vi "Edgertronic-:get_saved_settings copy.vi"(5 "Setup":T2={"URL"="130.64.16.195", "remote port"=80, "mode (standard)"=enum."Standard"}) -> (0 "error out":errorcluster, 1 "Saved Settings:":T1={"Connection Information:"="", "Requested Genlock "="20140911165611", "Min Frame Clocks "="20140911165611", "Is Seq Clk Freq "="20140911165611", "Pretrigger Frames "="20140911165611", "Duration "="20140911165611", "Overclock "="20140911165611", "Requested Horizontal "="20140911165611", "Frames "="20140911165611", "Requested Pretrigger "="20140911165611", "Words per Frame "="20140911165611", "Buffer End "="20140911165611", "Clocks per Frame  "="20140911165611", "Requested Duration "="20140911165611", "Pretrigger "="20140911165611", "Post-trigger Frames "="20140911165611", "Vertical "="20140911165611", "Requested Vertical "="20140911165611", "Reqested Frame Rate "="20140911165611", "Frame Rate "="20140911165611", "Horizontal "="20140911165611", "Clocks per Exposure "="20140911165611", "Digital Gain "="20140911165611", "Exposure "="20140911165611", "Genlock "="20140911165611", "Analog Gain "="20140911165611", "Subsample "="20140911165611", "Requested Exposure "="20140911165611", "Iso "="20140911165611", "Requested Overclock "="20140911165611", "Requested Subsample "="20140911165611", "Requested Iso"="20140911165611"}, 2 "data out":string="HTTP/1.0 200 OK\r\nContent-Type: text/html; charset=utf-8\r\nContent-Length: 313\r\nConnection: close\r\nDate: Tue, 16 Jun 2015 13:54:12 GMT\r\nServer: lighttpd/1.4.11 (edgertonic slow motion camera)\r\n\r\n{\"build_date\": \"20150112\", \"sw_build_date\": \"20140911165611\", \"fpga_initialized\": 1, \"hardware_revision\": 6, \"model_number\": 1, \"home_dir\": \"/home/root/ss-web\", \"ir_filter\": 1, \"mac_addr\": \"00:1B:C5:09:61:4D\", \"serial_console_enabled\": false, \"serial_number\": 333, \"fpga_version\": 70, \"hardware_configuration\": 1}")   [LabVIEW 2012]
doc: "This VI returns the values of the default settings."
panel:
  in  "GET Cmd":string="/get_saved_settings"
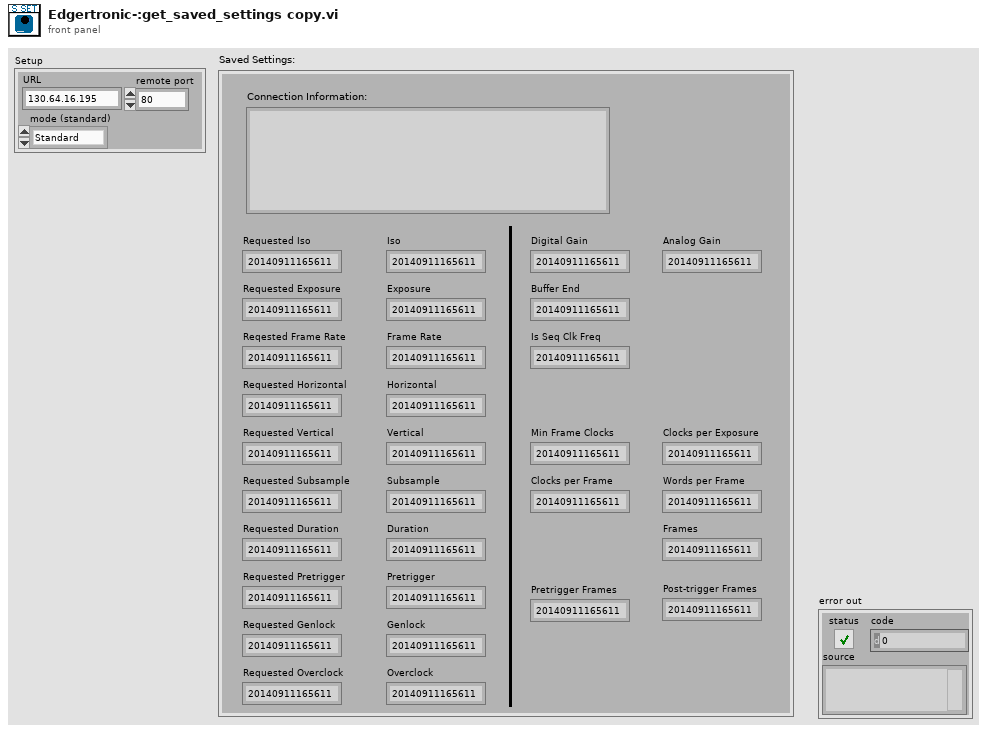
[diagram p1: front panel]
types:
  T1 = cluster{"Connection Information:":string, "Requested Genlock ":string, "Min Frame Clocks ":string, "Is Seq Clk Freq ":string, "Pretrigger Frames ":string, "Duration ":string, "Overclock ":string, "Requested Horizontal ":string, "Frames ":string, "Requested Pretrigger ":string, "Words per Frame ":string, "Buffer End ":string, "Clocks per Frame  ":string, "Requested Duration ":string, "Pretrigger ":string, "Post-trigger Frames ":string, "Vertical ":string, "Requested Vertical ":string, "Reqested Frame Rate ":string, "Frame Rate ":string, "Horizontal ":string, "Clocks per Exposure ":string, "Digital Gain ":string, "Exposure ":string, "Genlock ":string, "Analog Gain ":string, "Subsample ":string, "Requested Exposure ":string, "Iso ":string, "Requested Overclock ":string, "Requested Subsample ":string, "Requested Iso":string}
  T2 = cluster{"URL":string, "remote port":u16, "mode (standard)":enum16{"Standard", "Buffered", "CRLF", "Immediate"}}
  T3 = cluster{"Parameter":string, "Parameter 2":string, "Parameter 3":string, "Parameter 4":string, "Parameter 5":string, "Parameter 6":string, "Parameter 7":string, "Parameter 8":string, "Parameter 9":string, "Parameter 10":string, "Parameter 11":string, "Parameter 12":string, "Parameter 13":string, "Parameter 14":string, "Parameter 15":string, "Parameter 16":string, "Parameter 17":string, "Parameter 18":string, "Parameter 19":string, "Parameter 20":string, "Parameter 21":string, "Parameter 22":string, "Parameter 23":string, "Parameter 24":string, "Parameter 25":string, "Parameter 26":string, "Parameter 27":string, "Parameter 28":string, "Parameter 29":string, "Parameter 30":string, "Parameter 31":string, string, string, string, string, string}
  T4 = cluster{"[0]":string, "[1]":string, "[2]":string, "[3]":string, "[4]":string, "[5]":string, "[6]":string, "[7]":string, "[8]":string, "[9]":string, "[10]":string, "[11]":string, "[12]":string, "[13]":string, "[14]":string, "[15]":string, "[16]":string, "[17]":string, "[18]":string, "[19]":string, "[20]":string, "[21]":string, "[22]":string, "[23]":string, "[24]":string, "[25]":string, "[26]":string, "[27]":string, "[28]":string, "[29]":string, "[30]":string, "[31]":string, "[32]":string, "[33]":string, "[34]":string, "[35]":string}
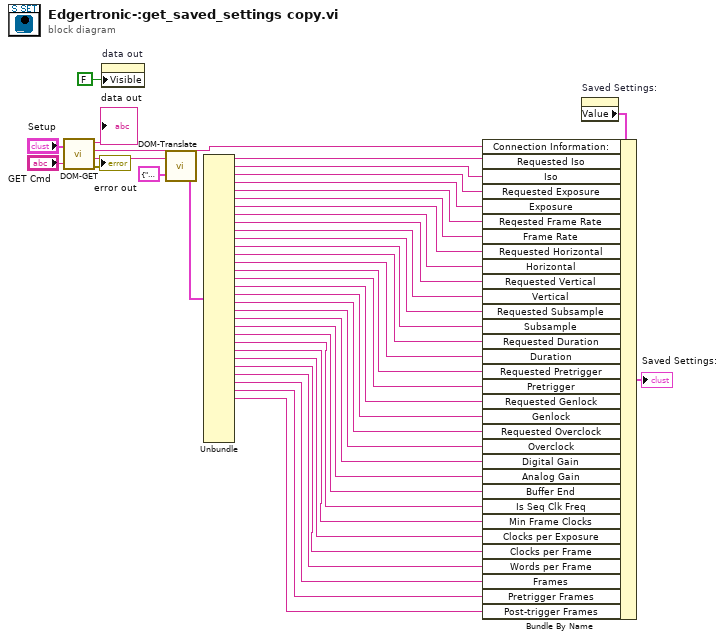
[diagram p0: block diagram]
diagram:
  n1 = call <userlib>:"DOM-GET.vi"("Setup"="Setup", "GET Command"="GET Cmd") -> ("Data Out from Camera"=→"data out":string, "Connection Information"=w36:string, "Value String"=w35:string, "error out"=→"error out":errorcluster)
  n2 = property on="data out" class="Str"("Visible"=FALSE) -> ()  [unwired: 2 in, 2 out]
  n3 = call <userlib>:"DOM-Translate.vi"("Parameter Cluster in"=T3 {"Parameter"="requested_iso", "Parameter 2"="iso", "Parameter 3"="requested_exposure", "Parameter 4"="exposure", "Parameter 5"="requested_frame_rate", "Parameter 6"="frame_rate", "Parameter 7"="requested_horizontal", "Parameter 8"="horizontal", "Parameter 9"="requested_vertical", "Parameter 10"="vertical", "Parameter 11"="requested_subsample", "Parameter 12"="subsample", "Parameter 13"="requested_duration", "Parameter 14"="duration", "Parameter 15"="requested_pretrigger", "Parameter 16"="pretrigger", "Parameter 17"="requested_genlock", "Parameter 18"="genlock", "Parameter 19"="requested_overclock", "Parameter 20"="overclock", "Parameter 21"="digital_gain", "Parameter 22"="analog_gain", "Parameter 23"="buffer_end", "Parameter 24"="is_seq_clk_freq", "Parameter 25"="min_frame_clocks", "Parameter 26"="clocks_per_exposure", "Parameter 27"="clocks_per_frame", "Parameter 28"="words_per_frame", "Parameter 29"="frames", "Parameter 30"="pretrigger_frames", "Parameter 31"="posttrigger_frames", "", "", "", "", ""}, "Value Data in"=w35) -> ("Value Cluster out"=w33:T4)
  n4 = Unbundle(w33) -> ("[0]"=w31:string, "[1]"=w30:string, "[2]"=w29:string, "[3]"=w28:string, "[4]"=w27:string, "[5]"=w26:string, "[6]"=w25:string, "[7]"=w24:string, "[8]"=w23:string, "[9]"=w22:string, "[10]"=w21:string, "[11]"=w20:string, "[12]"=w19:string, "[13]"=w18:string, "[14]"=w17:string, "[15]"=w16:string, "[16]"=w15:string, "[17]"=w14:string, "[18]"=w13:string, "[19]"=w12:string, "[20]"=w11:string, "[21]"=w10:string, "[22]"=w9:string, "[23]"=w8:string, "[24]"=w7:string, "[25]"=w6:string, "[26]"=w5:string, "[27]"=w4:string, "[28]"=w3:string, "[29]"=w2:string, "[30]"=w1:string)  [unwired: 5 out]
  n5 = property on="Saved Settings:" class="Clust (strict)"() -> ("Value"=w32:T1)  [unwired: 2 in, 2 out]
  n6 = Bundle By Name(cluster=w32, "Connection Information:"=w36, "Requested Iso"=w31, "Iso"=w30, "Requested Exposure"=w29, "Exposure"=w28, "Reqested Frame Rate"=w27, "Frame Rate"=w26, "Requested Horizontal"=w25, "Horizontal"=w24, "Requested Vertical"=w23, "Vertical"=w22, "Requested Subsample"=w21, "Subsample"=w20, "Requested Duration"=w19, "Duration"=w18, "Requested Pretrigger"=w17, "Pretrigger"=w16, "Requested Genlock"=w15, "Genlock"=w14, "Requested Overclock"=w13, "Overclock"=w12, "Digital Gain"=w11, "Analog Gain"=w10, "Buffer End"=w9, "Is Seq Clk Freq"=w8, "Min Frame Clocks"=w7, "Clocks per Exposure"=w6, "Clocks per Frame"=w5, "Words per Frame"=w4, "Frames"=w3, "Pretrigger Frames"=w2, "Post-trigger Frames"=w1) -> (→"Saved Settings:":T1)
